vi "HapticSTM_rawspeed2.vi"() -> ()   [LabVIEW 2019]
uses:
  SubVIs/GlobalClicksHeight_raw.vi
  <userlib>/HapticSTM/HapticSTM.lvlib
  <userlib>/Nanonis Prog Interface V5/Nanonis Prog Interface.lvlib
panel:
  in  "# Sample Points":i32=4096
  in  "Save":bool
  out "Fy 2":dbl format="%.1f"
  out "Fz 2":dbl format="%.1f"
  out "Fx 2":dbl format="%.1f"
  out "x 2":dbl format="%.1f"
  out "y 2":dbl format="%.1f"
  out "z 2":dbl format="%0.1f"
  in  "Hardness 2":dbl=0.7 format="%.1f"
  out "Clicks 2":i32
  out "H":dbl
  in  "START 2":bool
  in  "STOP 2":bool
  out "W":dbl
  out "Z Write":dbl format="%^.1e"
  out "Ox":dbl
  out "Oy":dbl
  out "Current (pA) 2":dbl format="%.1f"
  in  "Maximum (pA) 2":dbl=7000.0
  out "Scaled Force and Current":T1(graph)
  in  "Reset Clicks 2":bool
  out "Filtered Current (pA) 2":dbl format="%.1f"
  out "Button":bool
  in  "Mode":u16(ring) items=["Log w/ Exp Z", "Log w/ Lin Z", "Coulomb Force", "Lennard Jones", "r^6"]
  out "Raw and Scaled Z Positions":T2(graph)
  out "Setpoint (pA) 3":dbl
  in  "Depth (pA) 2":dbl=280.0
  in  "Planing? 2":bool
  in  "Scaling?":u16(ring) items=["Medium", "Large", "Small"]
  in  "Shift (in) 2":dbl format="%.1f"
  out "SeqString 2":string
  out "Seq 2":i32
  out "function return":i32
  in  "Z Write?":bool
  in  "Setpoint (pA) 2":dbl=100.0
  in  "Version? 2":bool=TRUE
  in  "Version?":bool=TRUE
  in  "Setpoint (pA)":dbl=100.0
  in  "Depth (pA)":dbl=280.0
  in  "Shift (in)":dbl format="%.1f"
  in  "Hardness":dbl=0.7 format="%.1f"
  out "Setpoint (pA)":dbl
  in  "Maximum (pA)":dbl=7000.0
  out "Filtered Current (pA)":dbl format="%.1f"
  out "Current (pA)":dbl format="%.1f"
  in  "Planing?":bool
  out "Fy":dbl format="%.1f"
  out "Fz":dbl format="%.1f"
  out "Fx":dbl format="%.1f"
  out "x":dbl format="%.1f"
  out "y":dbl format="%.1f"
  out "z":dbl format="%0.1f"
  in  "Reset Clicks":bool
  out "Clicks":i32
  in  "STOP":bool
  in  "START":bool
  out "Seq":i32
  out "SeqString":string
  # "Super Ultra Mega Haptic STM Controller 3000"
  # "Haptic Pen"
  # "Nanonis"
  # "Position"
  # "Z Controller"
  # "Force"
  # "Frame"
  # "Surface"
  # "Options"
  # "Addons"
  # "Test Data"
  # "Live"
  # "Current"
  # "No"
  # "Yes"
  # "Planing"
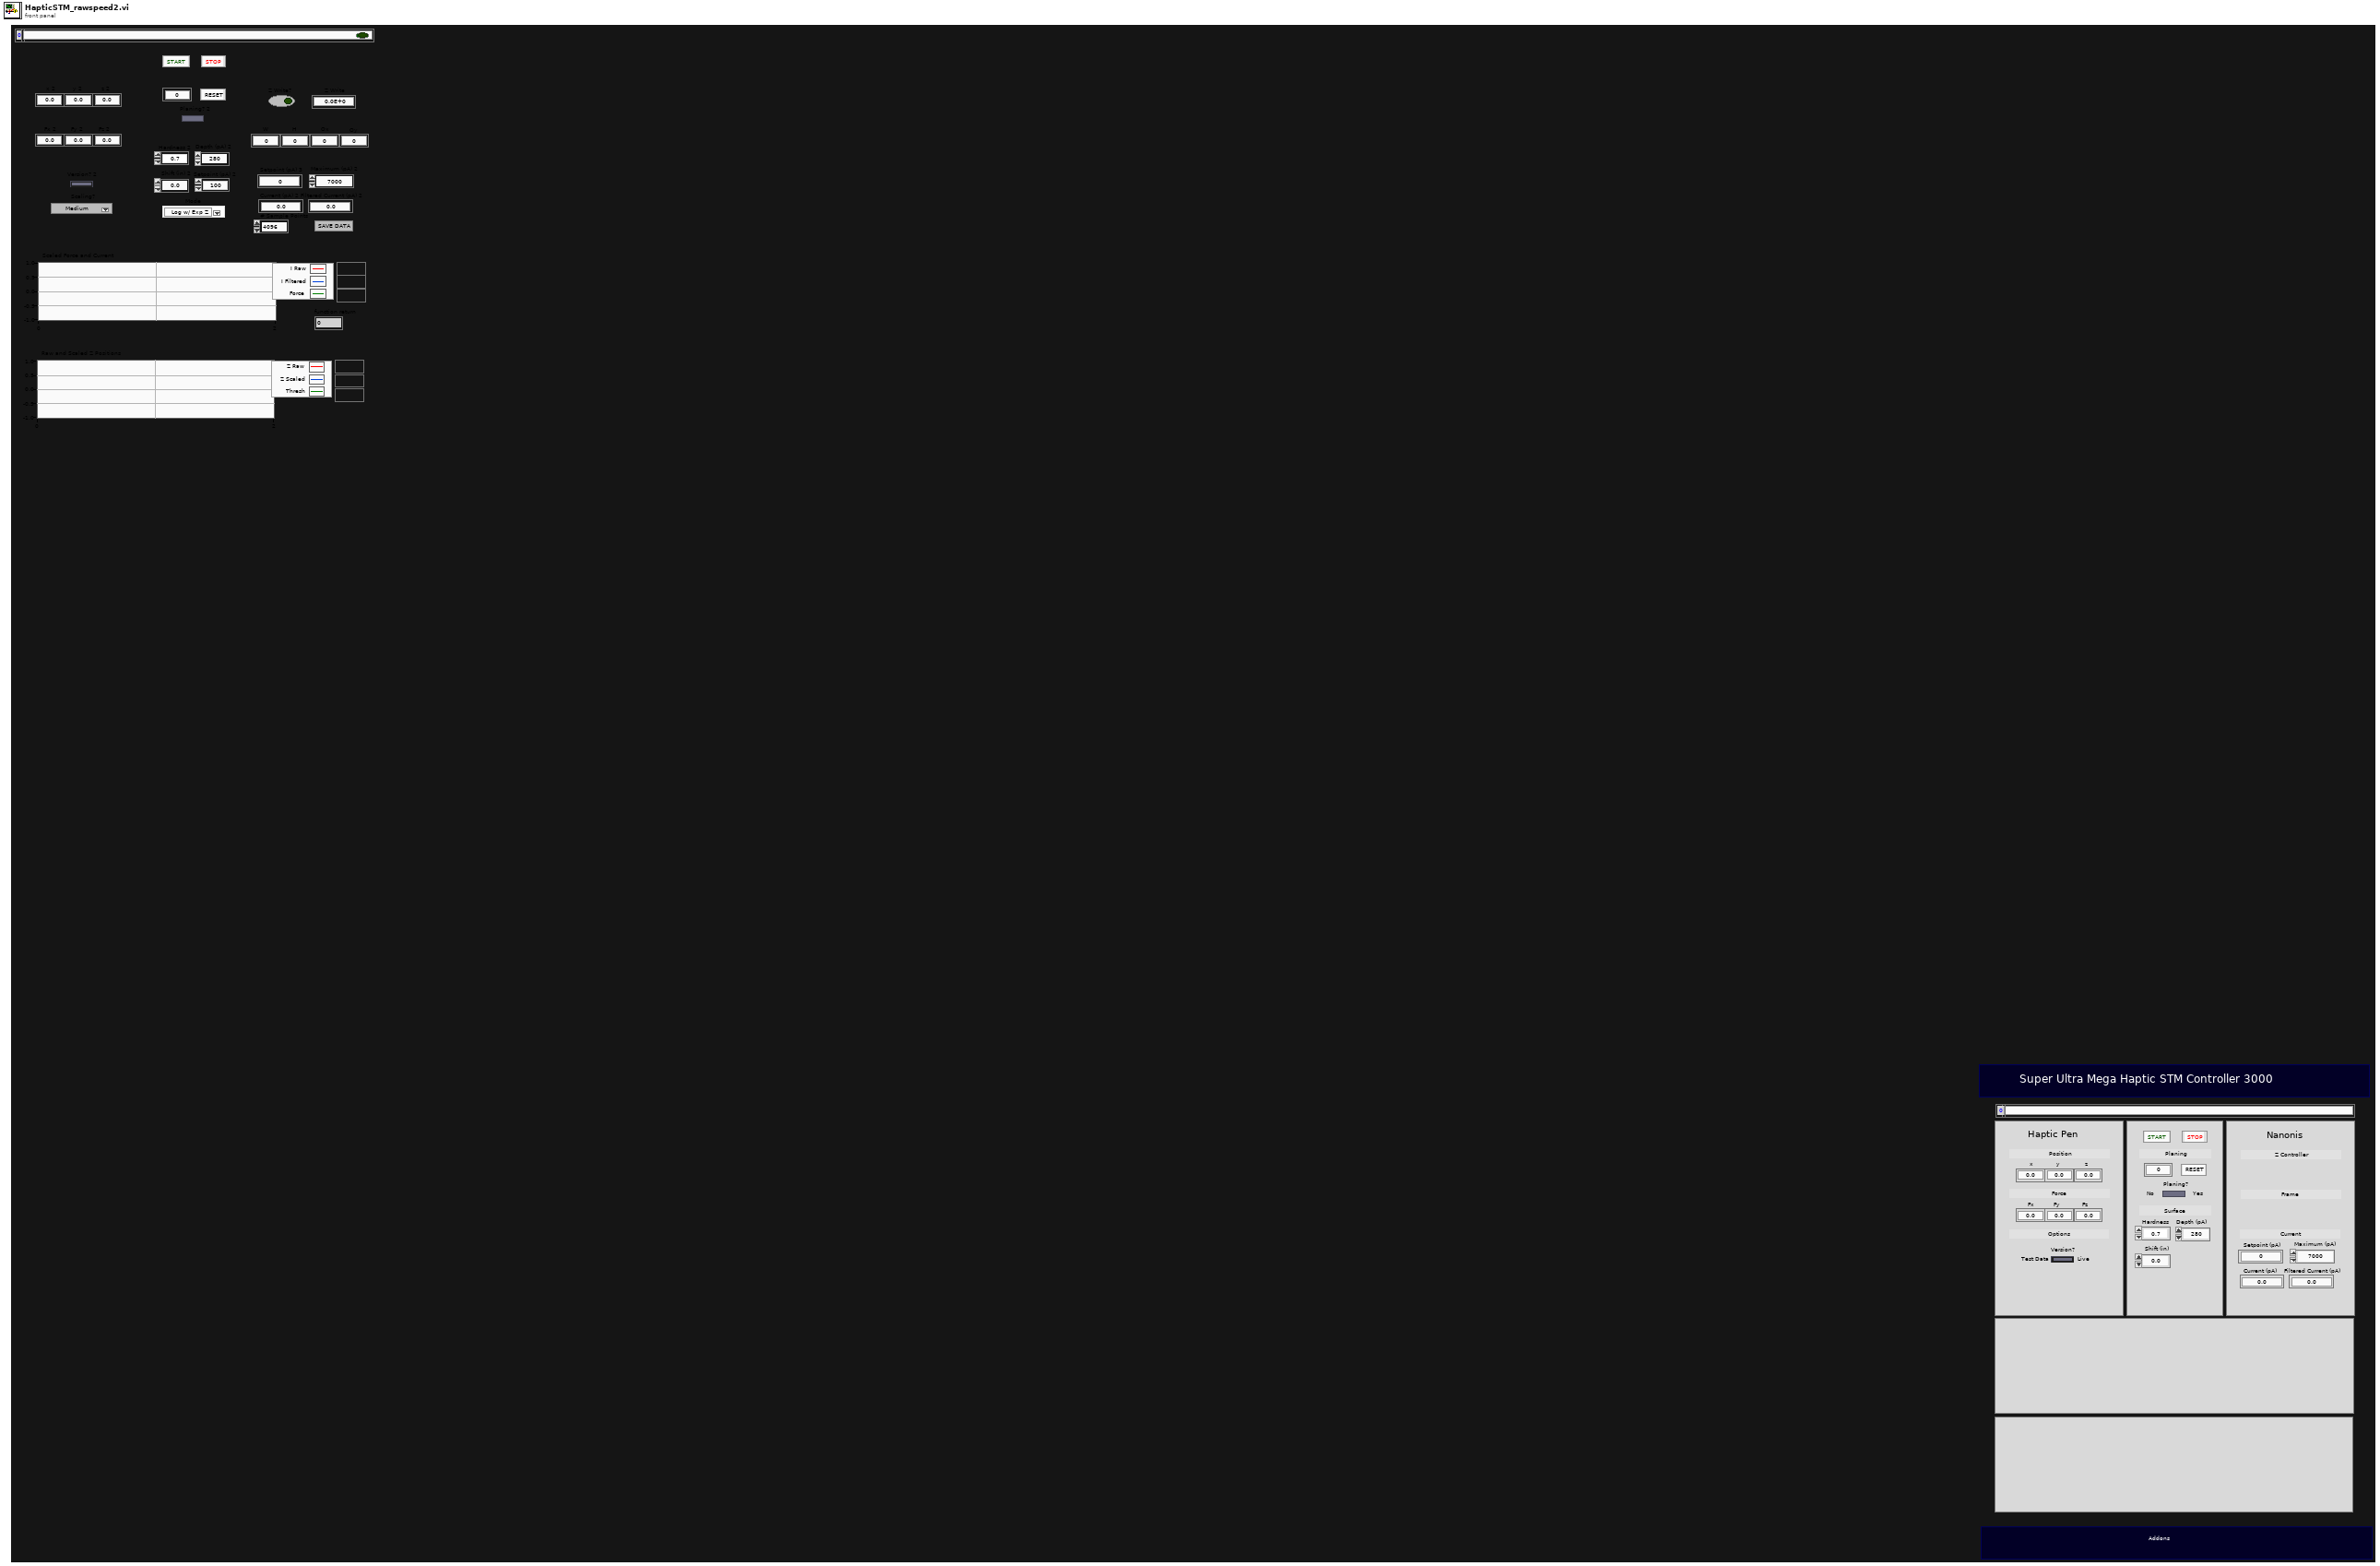
[diagram p1: front panel]
types:
  T1 = cluster{"Current (pA)":dbl, "Filtered Current (pA)":dbl, dbl}
  T2 = cluster{dbl, "function return":dbl, "function return":dbl}
  T3 = cluster{"Size (m)":cluster{"Width":sgl, "Height":sgl}, "Center coordinates (m)":cluster{"Xc":sgl, "Yc":sgl}}
  T4 = cluster{"Z Raw":dbl, "Z scaled":dbl, "threshhold":dbl}
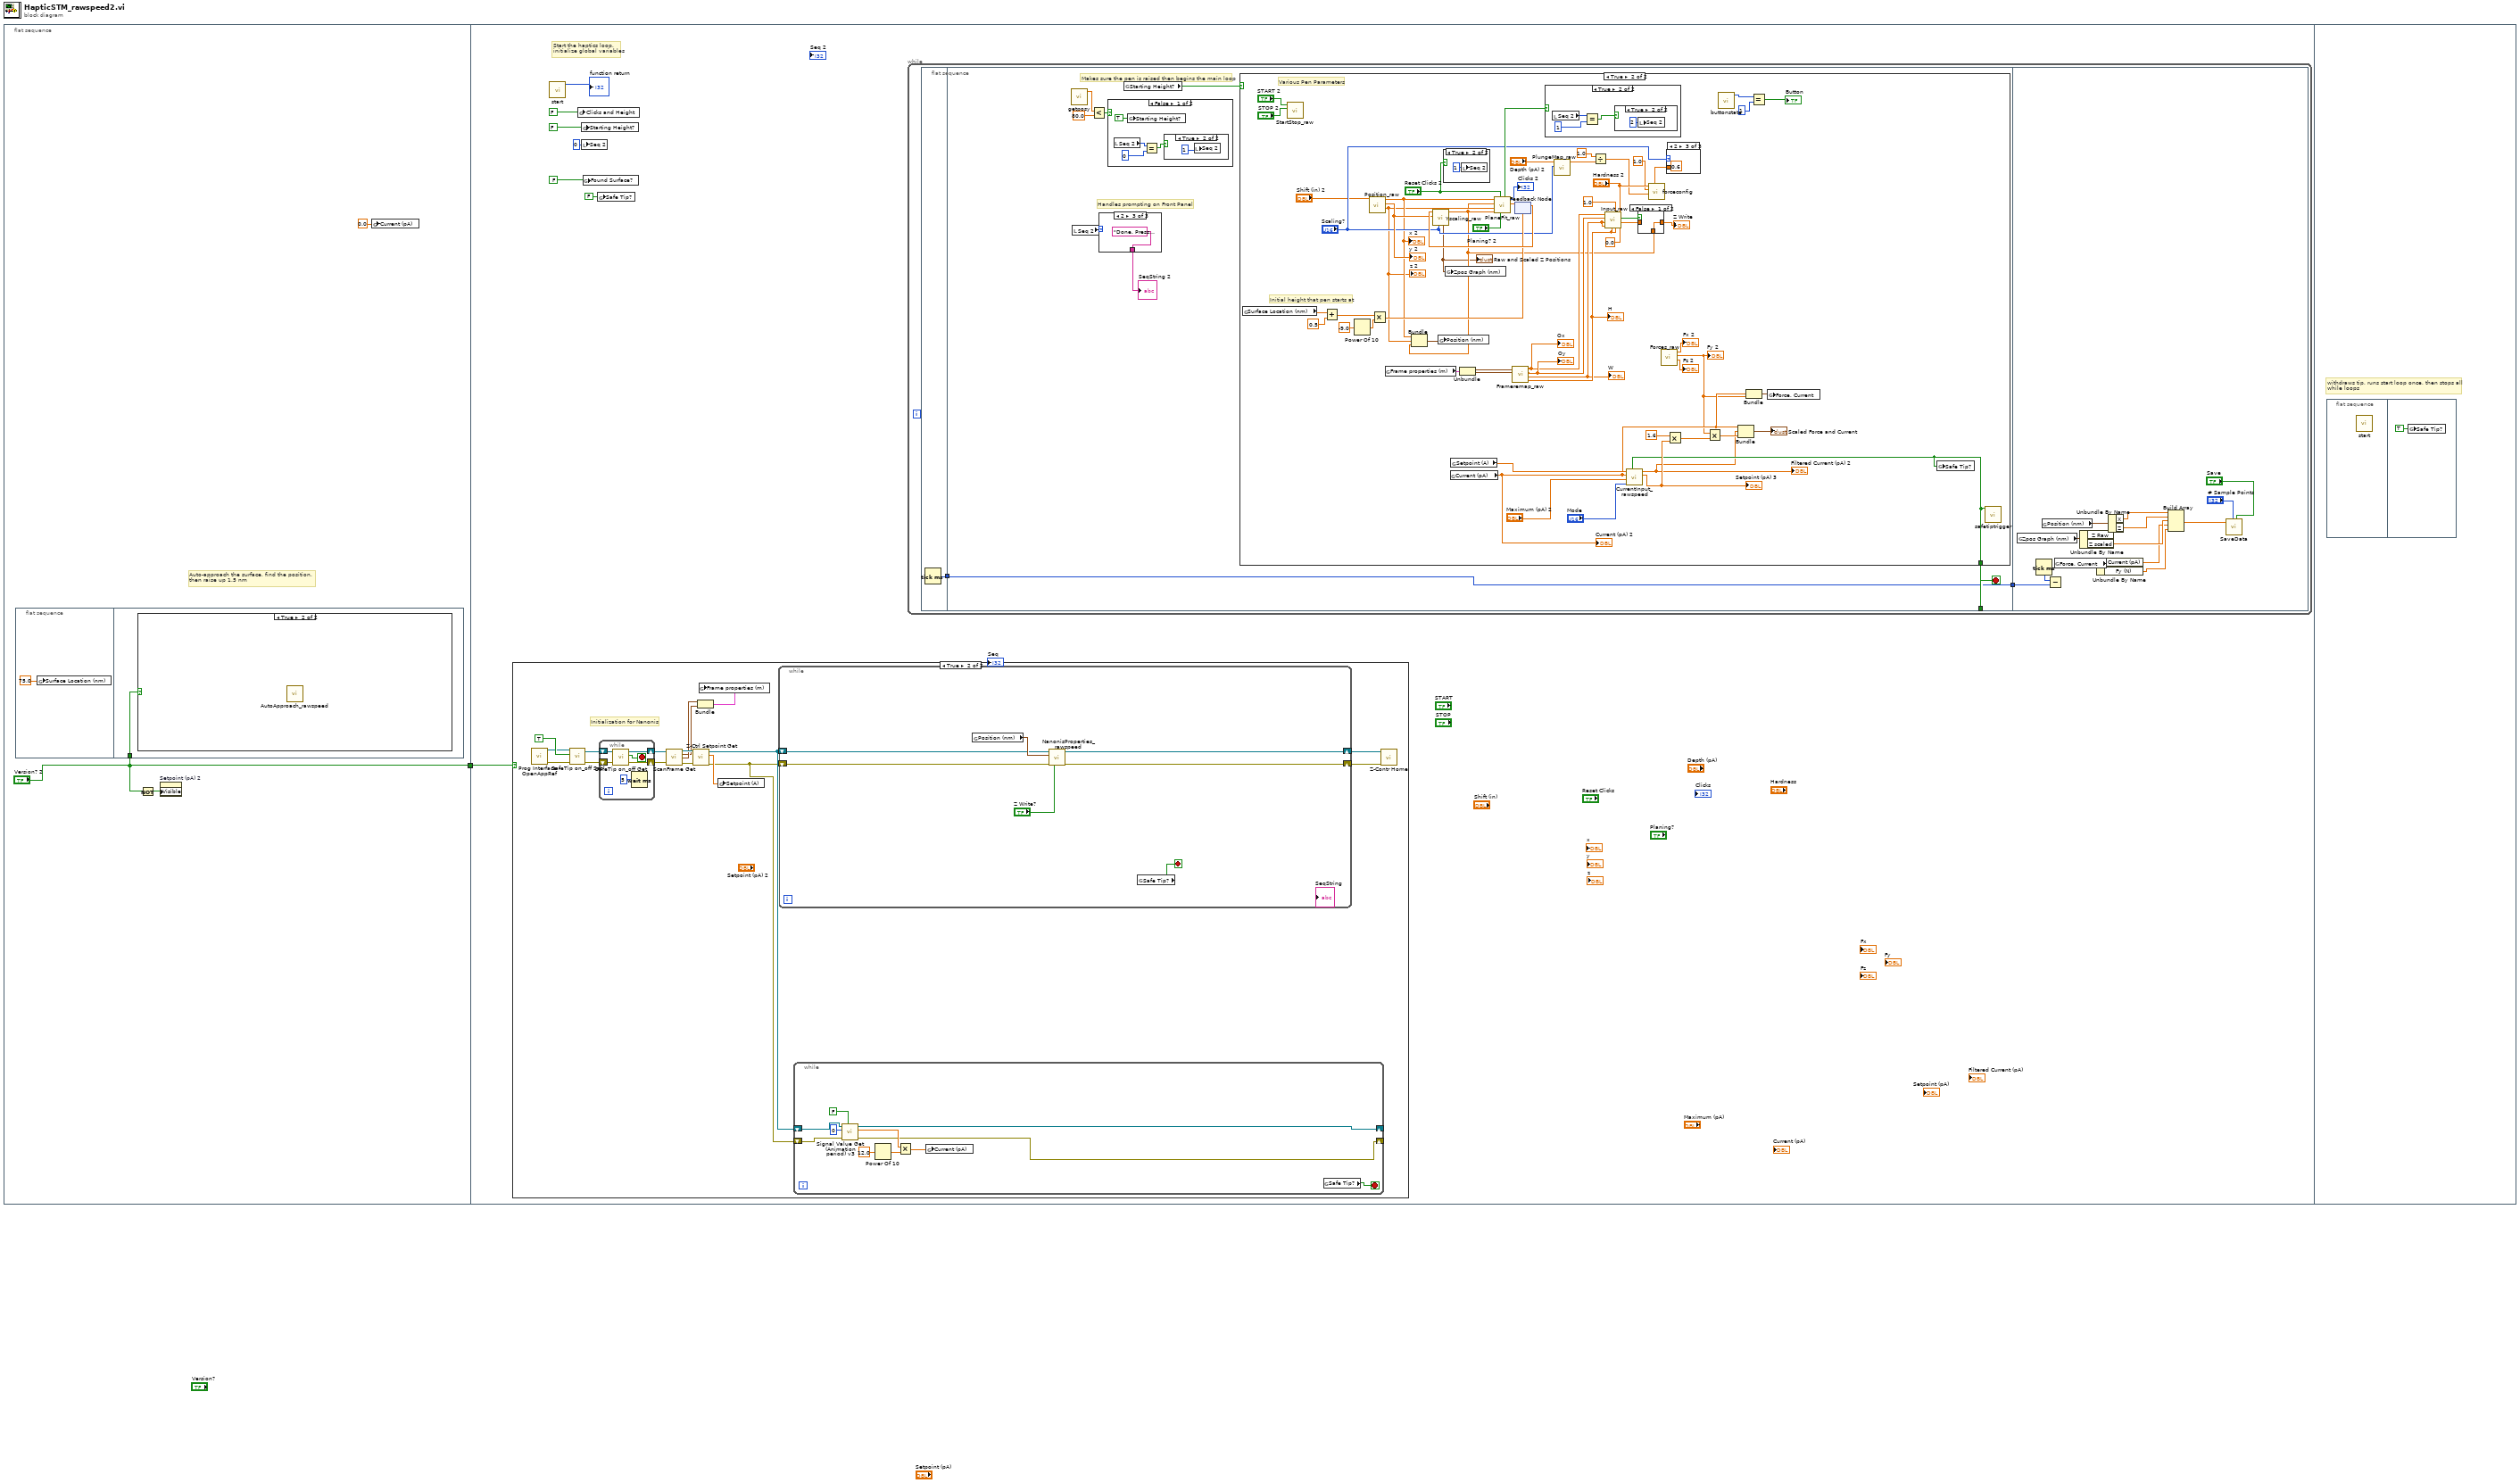
[diagram p0: block diagram]
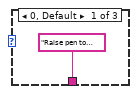
[diagram p4: hidden frame]
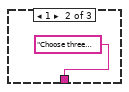
[diagram p5: hidden frame]
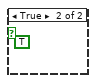
[diagram p7: hidden frame]
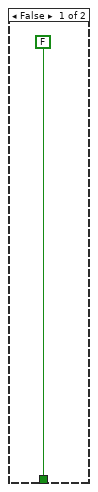
[diagram p8: hidden frame]
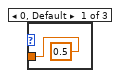
[diagram p9: hidden frame]
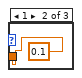
[diagram p10: hidden frame]
diagram:
  n1 = flat-sequence {
    tunnel: ["Version? 2"] -> w1
    tunnel: w1 -> [w7]
    frame #0 {
      # "Auto-approach the surface, find the position, \nthen raise up 1.5 nm"
      n2 = flat-sequence {
        tunnel: "Version? 2" -> [w6]
        frame #0 {
          n3 = global write "GlobalClicksHeight_raw.vi" "Surface Location (nm)"(75.0 ("Surface Location")) -> ()
        }
        frame #1 {
          n4 = case shown="True" w6 {
            frame False {
            }
            frame True {
              n5 = call "AutoApproach_rawspeed.vi"() -> ()  [unwired: 12 in]
            }
          }
        }
      }
      n6 = Not(x="Version? 2") -> (.not. x?=w3:bool)
      n7 = property on="Setpoint (pA) 2" class="DigNum (strict)"("Visible"=w3) -> ()  [unwired: 2 in, 2 out]
      n8 = global write "GlobalClicksHeight_raw.vi" "Current (pA)"(0.0 ("Current (pA)")) -> ()
    }
    frame #1 {
      # "Start the haptics loop,\ninitialize global variables"
      n9 = case shown="True" w7 {
        frame False {
        }
        frame True {
          # "Initialization for Nanonis"
          n10 = call <userlib>:"Prog Interface - OpenAppRef.vi"() -> ("Error out"=w28:errorcluster, "Application reference"=w29:refnum<vi>)  [unwired: 6 in]
          n11 = call <userlib>:"SafeTip on_off Set.vi"("error in (no error)"=w28, "SafeTip ON/OFF"=TRUE, "Application ref in"=w29) -> ("error out"=w26:errorcluster, "Application ref out"=w27:refnum<vi>)  [unwired: 7 in]
          n12 = while {
            shift-right: [w44] -> w25
            shift-left: w27 -> [w46]
            shift-right: [w43] -> w24
            shift-left: w26 -> [w45]
            stop <- w47 stop-if-true
            n13 = call <userlib>:"SafeTip on_off Get.vi"("error in (no error)"=w45, "Application ref in"=w46) -> ("error out"=w43:errorcluster, "SafeTip on/off status"=w47:bool, "Application ref out"=w44:refnum<vi>)  [unwired: 7 in]
            n14 = Wait (ms)(milliseconds to wait=u32 5) -> ()  [unwired: 1 out]
          }
          n15 = call <userlib>:"ScanFrame Get.vi"("Application ref in"=w25, "error in (no error)"=w24) -> ("Application ref out"=w23:refnum<vi>, "Center coordinates (m)"=w16:cluster{"Xc":sgl, "Yc":sgl}, "Size (m)"=w17:cluster{"Width":sgl, "Height":sgl}, "error out"=w22:errorcluster)  [unwired: 9 in, 1 out]
          n16 = call <userlib>:"Z-Ctrl Setpoint Get.vi"("error in (no error)"=w22, "Application ref in"=w23) -> ("error out"=w14:errorcluster, "Z Controller setpoint"=w21:sgl, "Application ref out"=w15:refnum<vi>)  [unwired: 6 in]
          n17 = Bundle("Size (m)"=w17, "Center coordinates (m)"=w16) -> (w18:T3)  [unwired: 1 in]
          n18 = global write "GlobalClicksHeight_raw.vi" "Frame properties (m)"(w18) -> ()
          n19 = global write "GlobalClicksHeight_raw.vi" "Setpoint (A)"(w21) -> ()
          n20 = while {
            shift-right: [w48] -> w19
            shift-left: w14 -> [w50]
            shift-right: [w49] -> w20
            shift-left: w15 -> [w51]
            stop <- w54 stop-if-true
            n21 = global read "GlobalClicksHeight_raw.vi" "Position (nm)"() -> (w52:cluster{"X":dbl, "Z":dbl, "Y":dbl})
            n22 = call "NanonisProperties_rawspeed.vi"("Application ref in"=w51, "Position (nm)"=w52, "error in (no error)"=w50, "Z Write?"="Z Write?") -> ("Application ref out"=w49:refnum<vi>, "error out"=w48:errorcluster)  [unwired: 10 in]
            n23 = global read "GlobalClicksHeight_raw.vi" "Safe Tip?"() -> (w54:bool)
          }
          n24 = while {
            shift-right: [w32] -> _
            shift-left: w14 -> [w34]
            shift-right: [w33] -> _
            shift-left: w15 -> [w35]
            stop <- w41 stop-if-true
            n25 = call <userlib>:"Signal Value Get (Animation period) v3.vi"("Wait for newest data (F=False)"=FALSE, "error in (no error)"=w34, "Signal index (0-127)"=i8 0, "Application ref in"=w35) -> ("error out"=w32:errorcluster, "Signal value"=w36:sgl, "Application ref out"=w33:refnum<vi>)  [unwired: 4 in]
            n26 = Power Of 10(x=12.0) -> (10^x=w39:dbl)
            n27 = Multiply(x=w36, y=w39) -> (x*y=w38:dbl)
            n28 = global write "GlobalClicksHeight_raw.vi" "Current (pA)"(w38) -> ()
            n29 = global read "GlobalClicksHeight_raw.vi" "Safe Tip?"() -> (w41:bool)
          }
          n30 = call <userlib>:"Z-Contr Home.vi"("Error in (no error)"=w19, "Application ref in"=w20) -> ()  [unwired: 8 in, 2 out]
        }
      }
      n31 = call <userlib>:"start.vi"() -> ("function return"=→"function return":i32)  [unwired: 11 in]
      n32 = global write "GlobalClicksHeight_raw.vi" "Clicks and Height"(FALSE ("Clicks and Height")) -> ()
      n33 = global write "GlobalClicksHeight_raw.vi" "Starting Height?"(FALSE ("Clicks and Height")) -> ()
      n34 = local write "Seq 2"(0 ("Seq")) -> ()
      n35 = global write "GlobalClicksHeight_raw.vi" "Found Surface?"(FALSE ("Clicks and Height")) -> ()
      n36 = global write "GlobalClicksHeight_raw.vi" "Safe Tip?"(FALSE ("Safe Tip?")) -> ()
      n37 = while {
        stop <- w57 stop-if-true
        n38 = flat-sequence {
          tunnel: [w58] -> w56
          tunnel: [w60] -> w57
          tunnel: w56 -> [w59]
          tunnel: [w59] -> w55
          tunnel: w55 -> [w156]
          frame #0 {
            n39 = Tick Count (ms)() -> (millisecond timer value=w58:u32)
          }
          frame #1 {
            # "Makes sure the pen is raised then begins the main loop"
            # "Handles prompting on Front Panel"
            n40 = call <userlib>:"getposy.vi"() -> ("function return"=w66:dbl)  [unwired: 11 in]
            n41 = local read "Seq 2"() -> (w62:i32)
            n42 = Less?(x=w66, y=80.0) -> (x < y?=w64:bool)
            n43 = case shown="2" w62 {
              tunnel: ["Raise pen to begin." "Choose three points, then raise the arm to plane." "Done. Press 'STOP' to stop at anytime."] -> w61
              frame 0, Default {
              }
              frame 1 {
              }
              frame 2 {
              }
            }
            "SeqString 2" <- w61
            n44 = case shown="False" w64 {
              frame False {
                n45 = local read "Seq 2"() -> (w72:i32)
                n46 = global write "GlobalClicksHeight_raw.vi" "Starting Height?"(TRUE ("Starting Height?")) -> ()
                n47 = Equal?(x=w72, y=0) -> (x = y?=w70:bool)
                n48 = case shown="True" w70 {
                  frame False {
                  }
                  frame True {
                    n49 = local write "Seq 2"(1 ("Seq")) -> ()
                  }
                }
              }
              frame True {
                (unwired) TRUE ("Clicks and Height")
              }
            }
            n50 = global read "GlobalClicksHeight_raw.vi" "Starting Height?"() -> (w63:bool)
            n51 = case shown="True" w63 {
              tunnel: [FALSE ("Current Maxed?") w85] -> w60
              frame False {
              }
              frame True {
                # "Initial height that pen starts at"
                # "Various Pen Parameters"
                n52 = global read "GlobalClicksHeight_raw.vi" "Surface Location (nm)"() -> (w99:dbl)
                n53 = call "StartStop_raw.vi"("STOP"="STOP 2", "START"="START 2") -> ()  [unwired: 10 in]
                n54 = Add(x=w99, y=0.5) -> (x+y=w96:dbl)
                n55 = Power Of 10(x=-9.0) -> (10^x=w95:dbl)
                n56 = call "Position_raw.vi"("Shift"="Shift (in) 2") -> ("Z"=w88:dbl, "Y"=w124:dbl, "X"=w89:dbl)  [unwired: 8 in]
                "x 2" <- w89
                "y 2" <- w124
                "z 2" <- w88
                n57 = Multiply(x=w96, y=w95) -> (x*y=w97:dbl)
                n58 = global read "GlobalClicksHeight_raw.vi" "Frame properties (m)"() -> (w84:cluster{cluster{dbl, dbl}, cluster{dbl, dbl}})
                n59 = case shown="True" "Reset Clicks 2" {
                  frame False {
                  }
                  frame True {
                    n60 = local write "Seq 2"(1 ("Seq")) -> ()
                  }
                }
                n61 = global read "GlobalClicksHeight_raw.vi" "Current (pA)"() -> (w79:dbl)
                "Current (pA) 2" <- w79
                n62 = global read "GlobalClicksHeight_raw.vi" "Setpoint (A)"() -> (w86:dbl)
                n63 = Unbundle(w84) -> (w83:cluster{dbl, dbl}, w82:cluster{dbl, dbl})
                n64 = call "Frameremap_raw.vi"("Frame Origin (m)"=w82, "Frame Size (m)"=w83) -> ("FH (nm)"=w109:dbl, "FW (nm)"=w108:dbl, "Z Origin (nm)"=w107:dbl, "X Origin (nm)"=w106:dbl)  [unwired: 6 in]
                "H" <- w109
                "W" <- w108
                "Ox" <- w106
                "Oy" <- w107
                n65 = feedback #1(w97) -> (w128:dbl)
                n66 = call "Yscaling_raw.vi"("Scaling?"="Scaling?", "Y"=w124, "Plane Height (m)"=w128) -> ("y scaled (m)"=w87:dbl, "Zpos Graph (nm)"=w77:T2)  [unwired: 7 in]
                "Raw and Scaled Z Positions" <- w77
                n67 = Bundle("X"=w89, "Z"=w88, "y scaled (m)"=w87) -> (w90:cluster{"X":dbl, "Z":dbl, "y scaled (m)":dbl})  [unwired: 1 in]
                n68 = global write "GlobalClicksHeight_raw.vi" "Position (nm)"(w90) -> ()
                n69 = global write "GlobalClicksHeight_raw.vi" "Zpos Graph (nm)"(w77) -> ()
                n70 = call "PlaneFit_raw.vi"("Planing y/n?"="Planing? 2", "Reset Clicks"="Reset Clicks 2", "Y PEN"=w87, "Z"=w88, "Nano Z"=w87, "X"=w89) -> ("Plane Height (m)"=w129:dbl, "Clicks"=→"Clicks 2":i32, "Planing Done?"=w118:bool)  [unwired: 3 in]
                n71 = feedback-in #1(w129) -> ()
                n72 = case shown="True" w118 {
                  frame False {
                  }
                  frame True {
                    n73 = local read "Seq 2"() -> (w143:i32)
                    n74 = Equal?(x=w143, y=1) -> (x = y?=w141:bool)
                    n75 = case shown="True" w141 {
                      frame False {
                      }
                      frame True {
                        n76 = local write "Seq 2"(2 ("Seq")) -> ()
                      }
                    }
                  }
                }
                n77 = call "PlungeMap_raw.vi"("Scaling?"="Scaling?", "Input (pA)"="Depth (pA) 2") -> ("output"=w100:dbl)  [unwired: 9 in]
                n78 = Divide(x=1.0, y=w100) -> (x/y=w110:dbl)
                n79 = call "Input_raw.vi"("Current * 10^input"=0.0, "Sensitivity"="Hardness 2", "Scopez"=w109, "Drag"=1.0, "FH"=w109, "FW"=w108, "Scopex"=w108, "Z origin"=w107, "X origin"=w106) -> ("Scaled Current"=w112:dbl, "feedback"=w114:bool)  [unwired: 1 in]
                n80 = call "CurrentInput_rawspeed.vi"("Mode"="Mode", "Maximum (pA)"="Maximum (pA) 2", "Current (pA)"=w79, "Setpoint (A)"=w86) -> ("Setpoint (pA)"=w102:dbl, "Filtered Current (pA)"=w78:dbl, "Safetip?"=w85:bool)  [unwired: 5 in]
                "Filtered Current (pA) 2" <- w78
                "Setpoint (pA) 3" <- w102
                n81 = case shown="False" w114 {
                  tunnel: [w138 w139] -> w113
                  tunnel: w112 -> [_ w139]
                  tunnel: w87 -> [w138 _]
                  frame False {
                  }
                  frame True {
                  }
                }
                "Z Write" <- w113
                n82 = call "Forces_raw.vi"() -> ("Fz"=→"Fz 2":dbl, "Fy"=w76:dbl, "Fx"=→"Fx 2":dbl)  [unwired: 9 in]
                "Fy 2" <- w76
                n83 = case shown="2" "Scaling?" {
                  tunnel: [0.5 0.1 0.6] -> w93
                  frame 0, Default {
                  }
                  frame 1 {
                  }
                  frame 2 {
                  }
                }
                n84 = call <userlib>:"forceconfig.vi"("spc"=w93, "c"=w110, "b"=1.0, "a"="Hardness 2") -> ()  [unwired: 8 in]
                n85 = Multiply(x=1.6 ("y"), y=w102) -> (x*y=w125:dbl)
                n86 = Multiply(x=w76, y=w125) -> (x*y=w127:dbl)
                n87 = call <userlib>:"buttonstate.vi"() -> ("function return"=w123:i32)  [unwired: 11 in]
                n88 = Bundle("Current (pA)"=w79, "Filtered Current (pA)"=w78, w127) -> (→"Scaled Force and Current":T1)  [unwired: 1 in]
                n89 = Bundle("Current (pA)"=w79, "Fy"=w76) -> (w80:cluster{"Current (pA)":dbl, "Fy":dbl})  [unwired: 1 in]
                n90 = Equal?(x=w123, y=1) -> (x = y?=→"Button":bool)
                n91 = global write "GlobalClicksHeight_raw.vi" "Force, Current"(w80) -> ()
                n92 = global write "GlobalClicksHeight_raw.vi" "Safe Tip?"(w85) -> ()
                n93 = call <userlib>:"safetiptrigger.vi"("triggered"=w85) -> ()  [unwired: 11 in]
              }
            }
          }
          frame #2 {
            n94 = global read "GlobalClicksHeight_raw.vi" "Zpos Graph (nm)"() -> (w152:T4)
            n95 = Tick Count (ms)() -> (millisecond timer value=w157:u32)
            n96 = global read "GlobalClicksHeight_raw.vi" "Position (nm)"() -> (w155:cluster{"X":dbl, "Z":dbl, "Y":dbl})
            n97 = Subtract(x=w157, y=w156) -> ()  [unwired: 1 out]
            n98 = global read "GlobalClicksHeight_raw.vi" "Force, Current"() -> (w150:cluster{"Current (pA)":dbl, "Fy (N)":dbl})
            n99 = Unbundle By Name(w152) -> ("Z scaled"=w151:dbl)  [unwired: 1 out]
            n100 = Unbundle By Name(w150) -> ("Current (pA)"=w149:dbl, "Fy (N)"=w148:dbl)
            n101 = Unbundle By Name(w155) -> ("X"=w154:dbl, "Z"=w153:dbl)
            n102 = Build Array(w154, w153, w151, w149, w148) -> (w147:dbl[])
            n103 = call "SaveData.vi"("Save"="Save", "# Sample Points"="# Sample Points", "Data"=w147) -> ()  [unwired: 9 in]
          }
        }
      }
    }
    frame #2 {
      # "withdraws tip, runs start loop once, then stops all\nwhile loops"
      n104 = flat-sequence {
        frame #0 {
          n105 = call <userlib>:"start.vi"() -> ()  [unwired: 11 in, 1 out]
        }
        frame #1 {
          n106 = global write "GlobalClicksHeight_raw.vi" "Safe Tip?"(TRUE ("Safe Tip?")) -> ()
        }
      }
    }
  }
